vi "Map Test to Tree.vi"(8 "error in (no error)":errorcluster, 11 "Test":T1={"Code"="", "Name"="", "Description"="", "Group"="", "IsGroup"=FALSE, "Tag"="", "Method"="", "Parrameter"="", "DataType"=enum."String", "Value"=variant, "Status"=enum."Pass", "LimitLo"=variant, "LimitHi"=variant, "StringMatch"="", "BooleanMatch"=FALSE, "DisplayFormat"="", "Units"="", "TestTime"=0.0}) -> (0 "error out":errorcluster, 1 "BG Colour":u32[](array[numeric]), 2 "Text Colour":u32[](array[numeric]), 3 "Text":string[](array[string]))   [LabVIEW 2022 SP3, in "TestView_Tree_Single.lvlib" / "TestView_Tree_Single.lvclass"]
uses:
  TestView_Tree_Single.lvclass
  Components/MES_Base.lvlibp/Controls/Test.ctl
  Components/MES_Base.lvlibp/MES_Base.lvclass
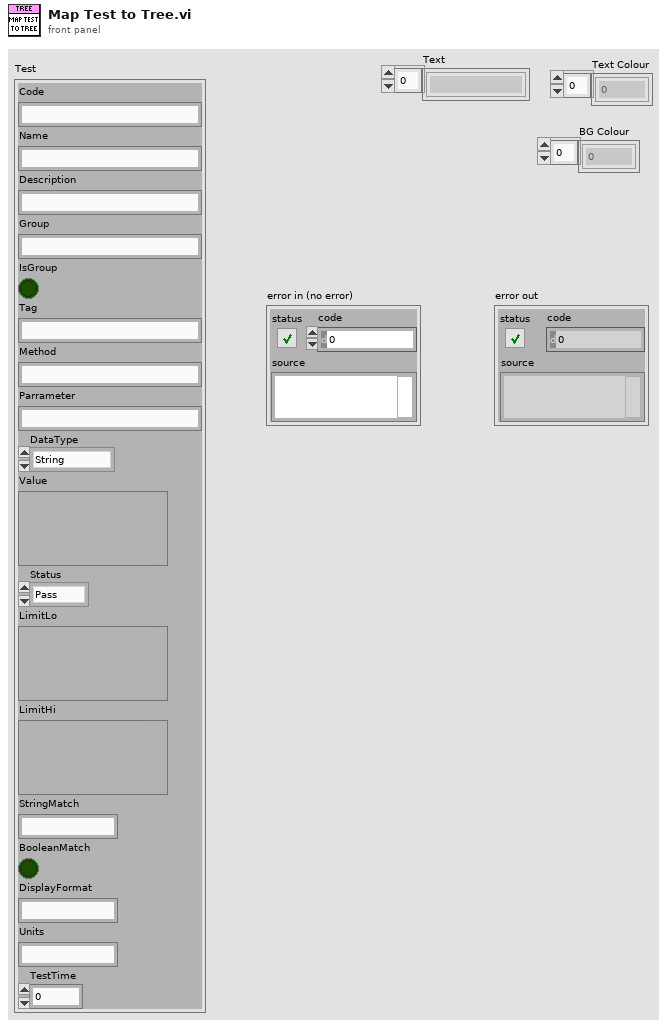
[diagram p1: front panel]
types:
  T1 = typedef "MES_Base.lvlibp/MES_Base.lvclass/Test.ctl" = cluster{"Code":string, "Name":string, "Description":string, "Group":string, "IsGroup":bool, "Tag":string, "Method":string, "Parrameter":string, "DataType":enum16{"NA", "String", "Boolean", "Int", "Dbl"}, "Value":variant, "Status":enum16{"Pending", "Pass", "Fail"}, "LimitLo":variant, "LimitHi":variant, "StringMatch":string, "BooleanMatch":bool, "DisplayFormat":string, "Units":string, "TestTime":dbl}
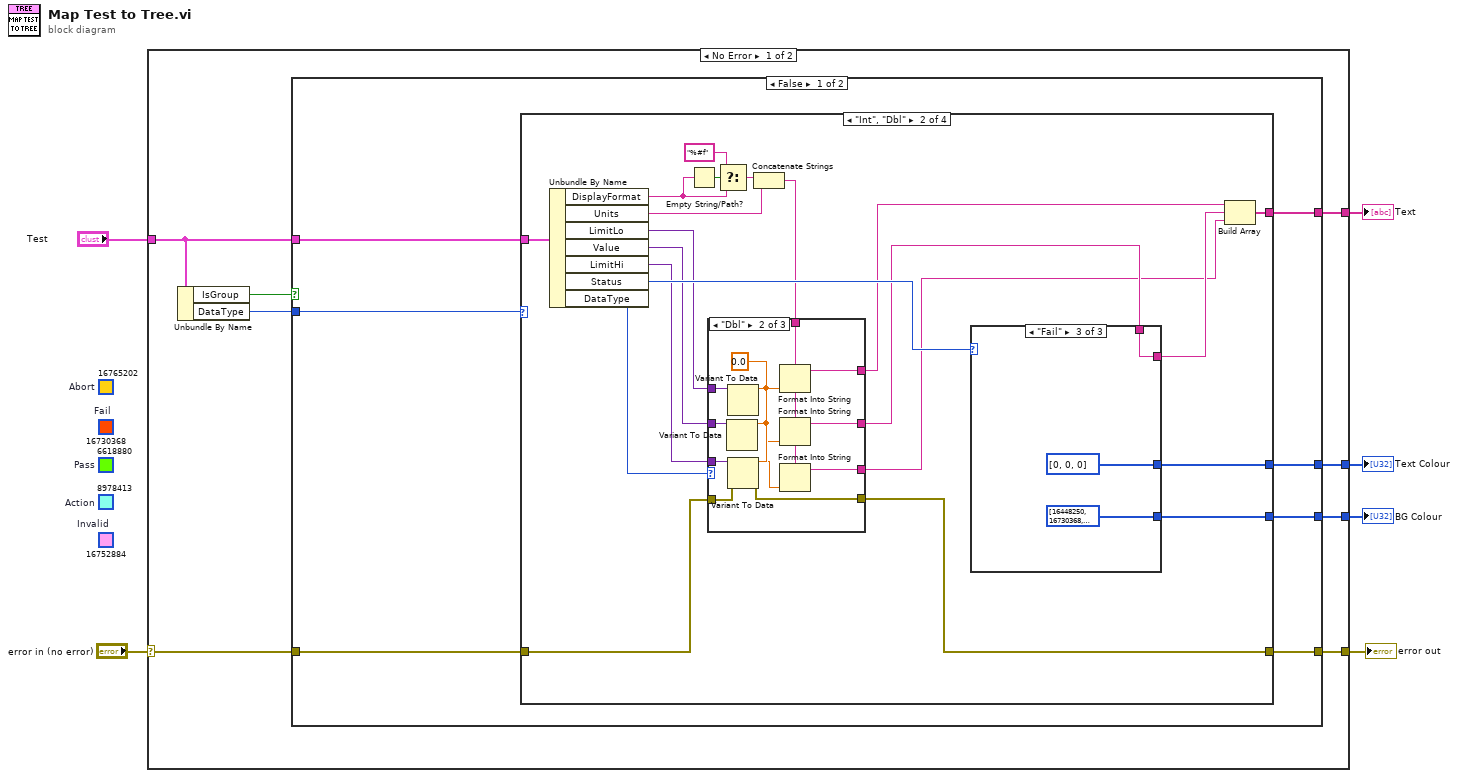
[diagram p0: block diagram]
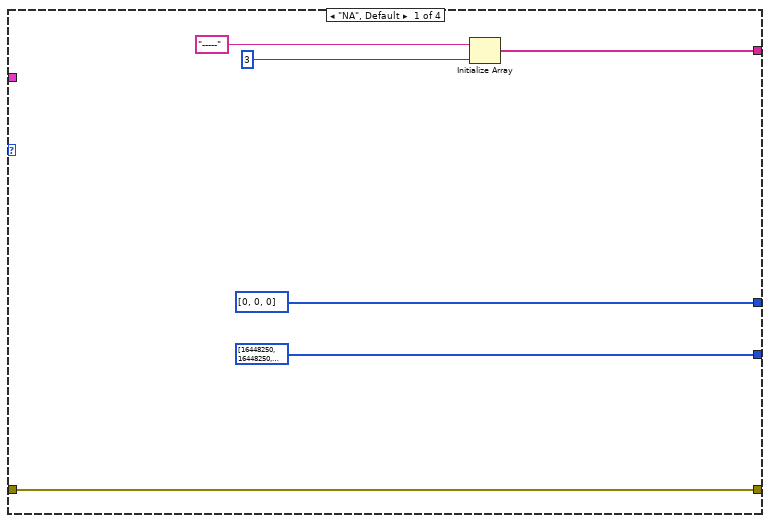
[diagram p2: hidden frame]
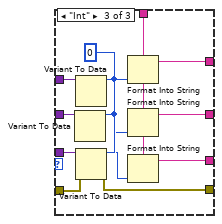
[diagram p4: hidden frame]
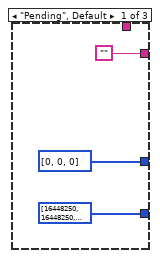
[diagram p5: hidden frame]
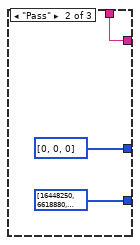
[diagram p6: hidden frame]
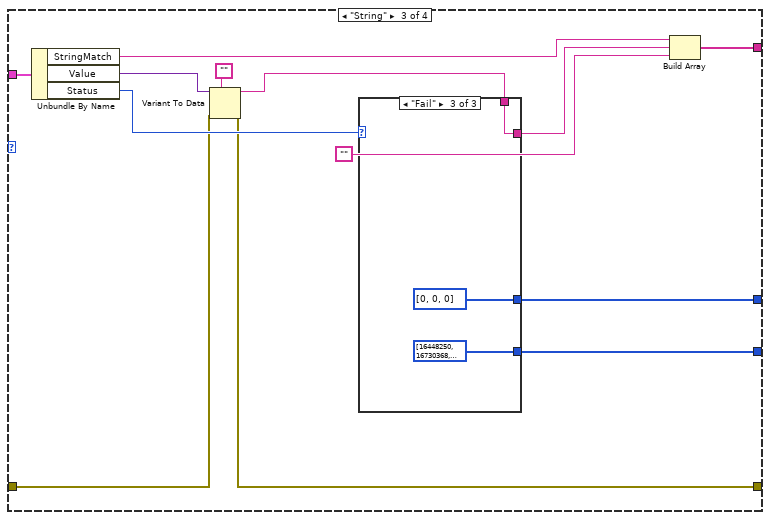
[diagram p7: hidden frame]
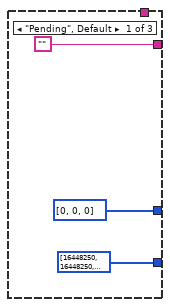
[diagram p8: hidden frame]
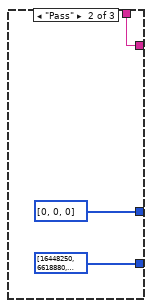
[diagram p9: hidden frame]
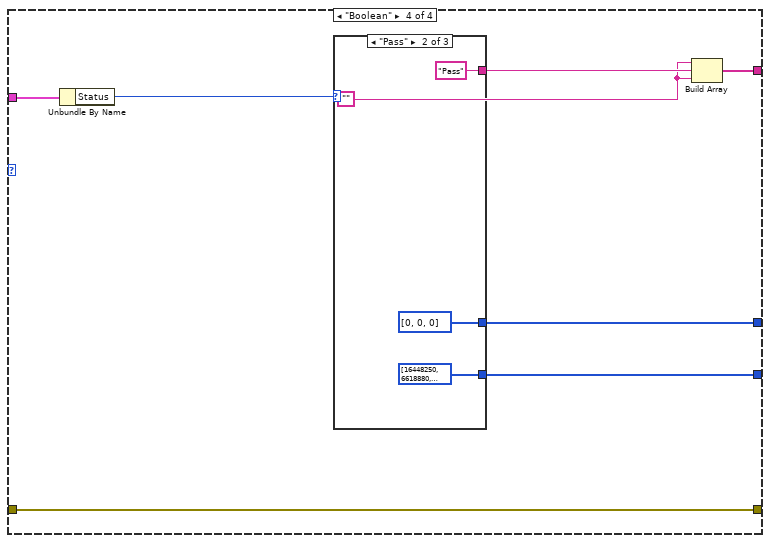
[diagram p10: hidden frame]
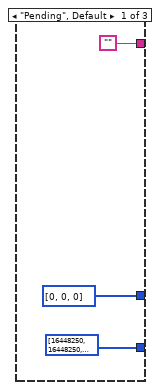
[diagram p11: hidden frame]
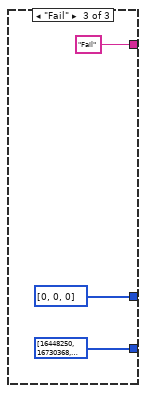
[diagram p12: hidden frame]
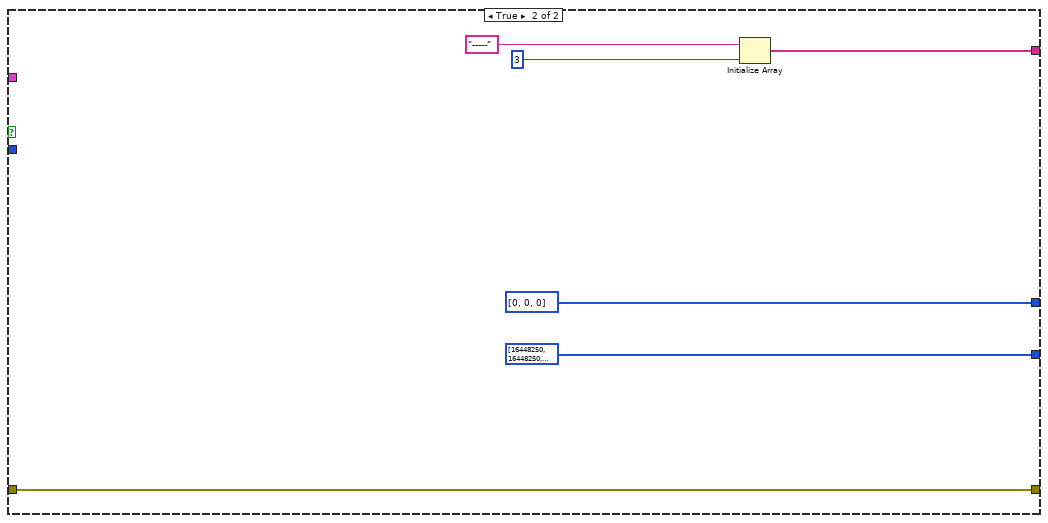
[diagram p13: hidden frame]
diagram:
  (unwired) u32 16752884  # Invalid
  (unwired) u32 8978413  # Action
  (unwired) u32 6618880  # Pass
  (unwired) u32 16730368  # Fail
  (unwired) u32 16765202  # Abort
  n1 = case shown="No Error" "error in (no error)" {
    selector: "error in (no error)" -> [w9 w130]
    tunnel: "Test" -> [w11 _]
    tunnel: [w14 _] -> w5
    tunnel: [w13 _] -> w4
    tunnel: [w12 _] -> w3
    tunnel: [w8 w130] -> w1
    frame No Error {
      n2 = Unbundle By Name(w11) -> ("IsGroup"=w7:bool, "DataType"=w10:enum16{"NA", "String", "Boolean", "Int", "Dbl"})
      n3 = case shown="False" w7 {
        tunnel: [w21 w127] -> w14
        tunnel: [w20 u32[] [0, 0, 0]] -> w13
        tunnel: [w19 u32[] [16448250, 16448250, 16448250]] -> w12
        tunnel: w11 -> [w18 _]
        tunnel: w10 -> [w15 _]
        tunnel: w9 -> [w17 w124]
        tunnel: [w16 w124] -> w8
        frame False {
          n4 = case shown="\"Int\", \"Dbl\"" w15 {
            tunnel: [w26 w47 w95 w114] -> w21
            tunnel: w18 -> [_ w48 w97 w113]
            tunnel: [u32[] [0, 0, 0] w39 w91 w109] -> w20
            tunnel: [u32[] [16448250, 16448250, 16448250] w38 w90 w108] -> w19
            tunnel: w17 -> [w22 w29 w86 w107]
            tunnel: [w22 w28 w85 w107] -> w16
            frame "NA", Default {
              n5 = Initialize Array("-----", 3 ("dimension size")) -> (w26:string[])
            }
            frame "Int", "Dbl" {
              n6 = Unbundle By Name(w48) -> ("DisplayFormat"=w42:string, "Units"=w44:string, "LimitLo"=w37:variant, "Value"=w36:variant, "LimitHi"=w35:variant, "Status"=w46:enum16{"Pending", "Pass", "Fail"}, "DataType"=w34:enum16{"NA", "String", "Boolean", "Int", "Dbl"})
              n7 = Empty String/Path?(string/path=w42) -> (empty?=w43:bool)
              n8 = Select(t="%#f" ("format string"), s=w43, f=w42) -> (s? t:f=w40:string)
              n9 = Concatenate Strings(w40, w44) -> (w33:string)
              n10 = case shown="\"Dbl\"" w34 {
                tunnel: w37 -> [_ w62 w75]
                tunnel: w36 -> [_ w61 w74]
                tunnel: w35 -> [_ w60 w73]
                tunnel: w33 -> [_ w57 w70]
                tunnel: [_ w54 w67] -> w32
                tunnel: [_ w53 w66] -> w31
                tunnel: [_ w52 w65] -> w30
                tunnel: w29 -> [w49 w51 w64]
                tunnel: [w49 w50 w63] -> w28
                frame "NA", Default {
                }
                frame "Dbl" {
                  w59 = 0.0
                  n11 = Variant To Data(type=w59, Variant=w61) -> (data=w56:dbl)  [unwired: 1 in, 1 out]
                  n12 = Variant To Data(type=w59, Variant=w62) -> (data=w58:dbl)  [unwired: 1 in, 1 out]
                  n13 = Variant To Data(error in=w51, type=w59, Variant=w60) -> (data=w55:dbl, error out=w50:errorcluster)
                  n14 = Format Into String(format string=w57, w58) -> (resulting string=w54:string)  [unwired: 2 in, 1 out]
                  n15 = Format Into String(format string=w57, w56) -> (resulting string=w53:string)  [unwired: 2 in, 1 out]
                  n16 = Format Into String(format string=w57, w55) -> (resulting string=w52:string)  [unwired: 2 in, 1 out]
                }
                frame "Int" {
                  w72 = 0
                  n17 = Variant To Data(type=w72, Variant=w74) -> (data=w69:i32)  [unwired: 1 in, 1 out]
                  n18 = Variant To Data(type=w72, Variant=w75) -> (data=w71:i32)  [unwired: 1 in, 1 out]
                  n19 = Variant To Data(error in=w64, type=w72, Variant=w73) -> (data=w68:i32, error out=w63:errorcluster)
                  n20 = Format Into String(format string=w70, w71) -> (resulting string=w67:string)  [unwired: 2 in, 1 out]
                  n21 = Format Into String(format string=w70, w69) -> (resulting string=w66:string)  [unwired: 2 in, 1 out]
                  n22 = Format Into String(format string=w70, w68) -> (resulting string=w65:string)  [unwired: 2 in, 1 out]
                }
              }
              n23 = case shown="\"Fail\"" w46 {
                tunnel: ["" w81 w84] -> w45
                tunnel: w31 -> [_ w81 w84]
                tunnel: [u32[] [0, 0, 0] u32[] [0, 0, 0] u32[] [0, 0, 0]] -> w39
                tunnel: [u32[] [16448250, 16448250, 16448250] u32[] [16448250, 6618880, 16448250] u32[] [16448250, 16730368, 16448250]] -> w38
                frame "Pending", Default {
                }
                frame "Pass" {
                }
                frame "Fail" {
                }
              }
              n24 = Build Array(w32, w45, w30) -> (w47:string[])
            }
            frame "String" {
              n25 = Unbundle By Name(w97) -> ("StringMatch"=w96:string, "Value"=w88:variant, "Status"=w93:enum16{"Pending", "Pass", "Fail"})
              n26 = Variant To Data(error in=w86, type="", Variant=w88) -> (data=w87:string, error out=w85:errorcluster)
              n27 = case shown="\"Fail\"" w93 {
                tunnel: ["" w103 w106] -> w92
                tunnel: w87 -> [_ w103 w106]
                tunnel: [u32[] [0, 0, 0] u32[] [0, 0, 0] u32[] [0, 0, 0]] -> w91
                tunnel: [u32[] [16448250, 16448250, 16448250] u32[] [16448250, 6618880, 16448250] u32[] [16448250, 16730368, 16448250]] -> w90
                frame "Pending", Default {
                }
                frame "Pass" {
                }
                frame "Fail" {
                }
              }
              n28 = Build Array(w96, w92, "") -> (w95:string[])
            }
            frame "Boolean" {
              w110 = ""
              n29 = Unbundle By Name(w113) -> ("Status"=w112:enum16{"Pending", "Pass", "Fail"})
              n30 = case shown="\"Pass\"" w112 {
                tunnel: ["" "Pass" "Fail"] -> w111
                tunnel: [u32[] [0, 0, 0] u32[] [0, 0, 0] u32[] [0, 0, 0]] -> w109
                tunnel: [u32[] [16448250, 16448250, 16448250] u32[] [16448250, 6618880, 16448250] u32[] [16448250, 16730368, 16448250]] -> w108
                frame "Pending", Default {
                }
                frame "Pass" {
                }
                frame "Fail" {
                }
              }
              n31 = Build Array(w110, w111, w110) -> (w114:string[])
            }
          }
        }
        frame True {
          n32 = Initialize Array("-----", 3 ("dimension size")) -> (w127:string[])
        }
      }
    }
    frame Error {
    }
  }
  "Text" <- w5
  "Text Colour" <- w4
  "BG Colour" <- w3
  "error out" <- w1
